vi "Module Loop.vi"(8 "error in (no error)":errorcluster, 11 "EStop Module in":refnum<class "EStop Module.lvclass">) -> (0 "error out":errorcluster, 3 "EStop Module out":refnum<class "EStop Module.lvclass">)   [LabVIEW 2020, in "VolatusControl.lvlib" / "EStop Module.lvclass"]
uses:
  EStop Module.lvclass
  C:/dev/lv20CE/relink/lv-volatus/Volatus/Module/Module.lvclass
  Volatus/Module/Module.lvclass
  Volatus/Module/Module.lvclass/Module.ctl
  <vilib>/Utility/error.llb/Error Cluster From Error Code.vi
  EStop Module.lvclass/EStop Module.ctl
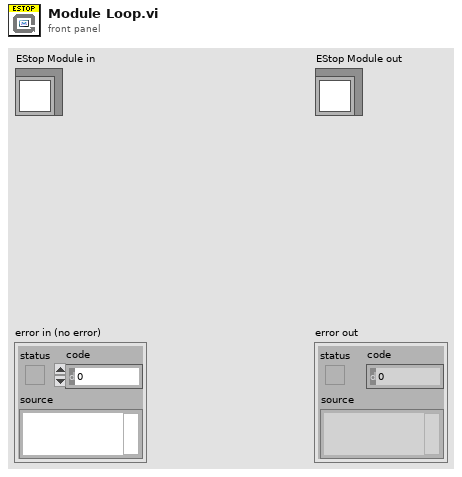
[diagram p1: front panel]
types:
  T1 = enum32{"Invalid", "Standard", "Closed", "Hidden", "Minimized", "Maximized"}
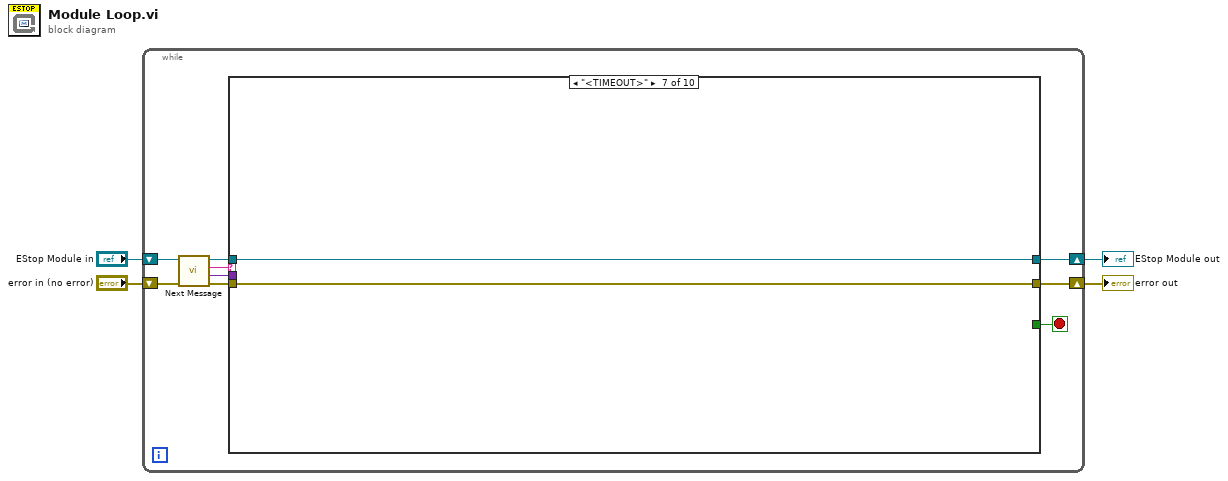
[diagram p0: block diagram]
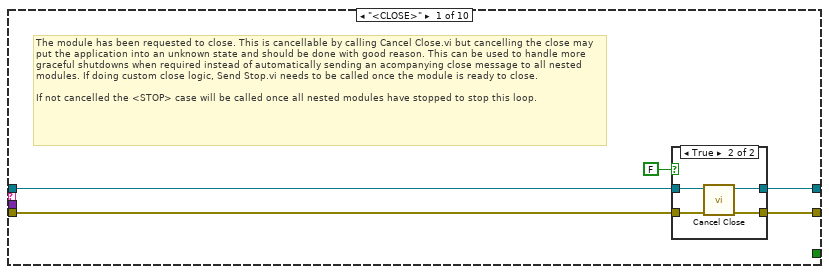
[diagram p2: hidden frame]
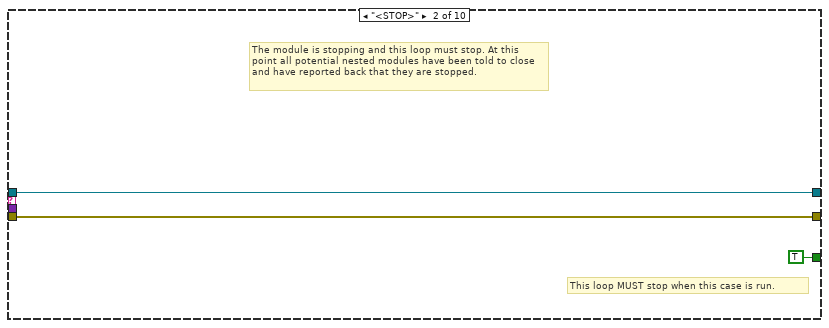
[diagram p4: hidden frame]
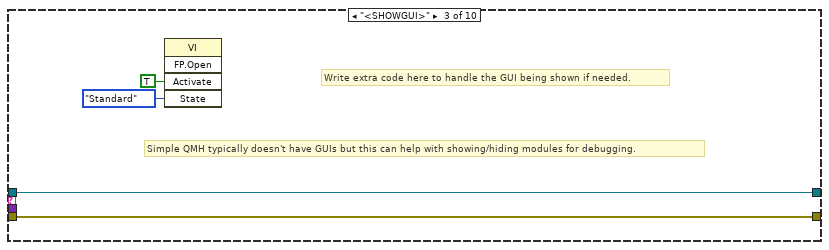
[diagram p5: hidden frame]
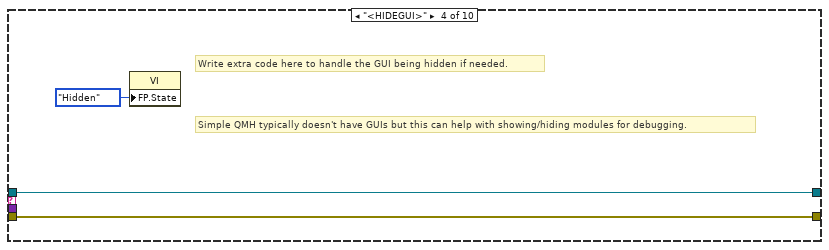
[diagram p6: hidden frame]
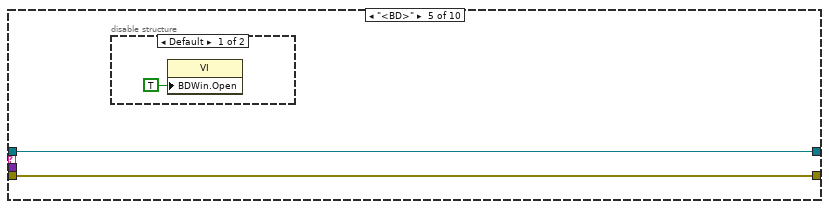
[diagram p7: hidden frame]
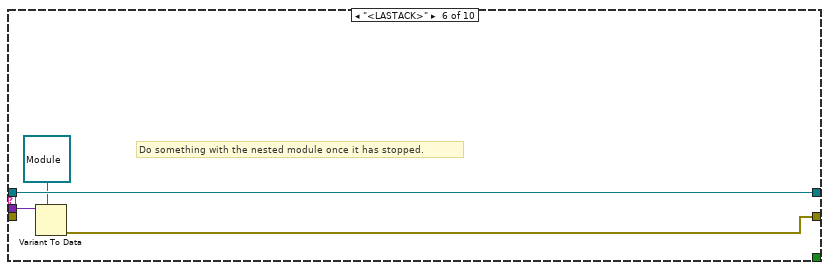
[diagram p9: hidden frame]
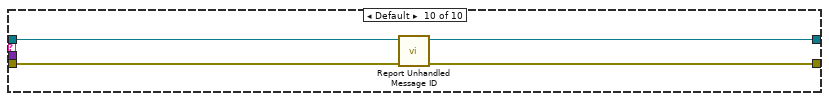
[diagram p12: hidden frame]
diagram:
  n1 = while {
    shift-right: [w8] -> w2
    shift-left: "EStop Module in" -> [w13]
    shift-right: [w7] -> w1
    shift-left: "error in (no error)" -> [w12]
    stop <- w6 stop-if-true
    n2 = call "Next Message.vi"("error in (no error)"=w12, "Module in"=w13) -> ("error out"=w11:errorcluster, "Data"=w5:variant, "ID"=w10:string, "Module out"=w9:refnum<class "EStop Module.lvclass">)  [unwired: 6 in]
    n3 = case shown="\"<TIMEOUT>\"" w10 {
      tunnel: w11 -> [w18 w26 w30 w33 w35 _ w42 w44 w46 w51]
      tunnel: w9 -> [w16 w27 w31 w34 w36 w41 w43 w45 w47 w49]
      tunnel: [w15 w27 w31 w34 w36 w41 w43 w45 w47 w48] -> w8
      tunnel: [w17 w26 w30 w33 w35 w38 w42 w44 w46 w50] -> w7
      tunnel: [_ TRUE _ _ _ _ _ _ _ _] -> w6
      tunnel: w5 -> [_ _ _ _ _ w40 _ _ _ _]
      frame "<CLOSE>" {
        # "The module has been requested to close. This is cancellable by calling Cancel Close.vi but cancelling the close may put the application into an unknown state and should be done with good reason. This can be used to handle more graceful shutdowns when required instead of automatically sending an acompanying close message to all nested modules. If doing custom close logic, Send Stop.vi needs to be called once the module is ready to close.\n\nIf not cancelled the <STOP> case will be called once all nested modules have stopped to stop this loop."
        n4 = case shown="True" FALSE {
          tunnel: w18 -> [w19 w24]
          tunnel: [w19 w23] -> w17
          tunnel: w16 -> [w20 w22]
          tunnel: [w20 w21] -> w15
          frame False {
          }
          frame True {
            n5 = call "Cancel Close.vi"("error in (no error)"=w24, "Module in"=w22) -> ("error out"=w23:errorcluster, "Module out"=w21:refnum<class "EStop Module.lvclass">)  [unwired: 8 in]
          }
        }
      }
      frame "<STOP>" {
        # "This loop MUST stop when this case is run."
        # "The module is stopping and this loop must stop. At this point all potential nested modules have been told to close and have reported back that they are stopped."
      }
      frame "<SHOWGUI>" {
        # "Simple QMH typically doesn't have GUIs but this can help with showing/hiding modules for debugging."
        # "Write extra code here to handle the GUI being shown if needed."
        n6 = invoke class="VI" method="FP.Open"("Activate"=TRUE ("Activate?"), "State"=T1."Standard") -> ()  [unwired: 3 in, 5 out]
      }
      frame "<HIDEGUI>" {
        # "Simple QMH typically doesn't have GUIs but this can help with showing/hiding modules for debugging."
        # "Write extra code here to handle the GUI being hidden if needed."
        n7 = property class="VI"("FP.State"=T1."Hidden" ("Front Panel Window:State")) -> ()  [unwired: 2 in, 2 out]
      }
      frame "<BD>" {
        n8 = disable-structure shown="Default" {
          frame condition #0 (active) {
            n9 = property class="VI"("BDWin.Open"=TRUE ("Block Diagram Window:Open")) -> ()  [unwired: 2 in, 2 out]
          }
          frame condition #1 {
          }
        }
      }
      frame "<LASTACK>" {
        # "Do something with the nested module once it has stopped."
        n10 = Variant To Data(type=refnum<class "Module.lvclass"> refnum ("Volatus:Module"), Variant=w40) -> (error out=w38:errorcluster)  [unwired: 1 in, 1 out]
      }
      frame "<TIMEOUT>" {
      }
      frame "Initialize" {
      }
      frame "EStop" {
      }
      frame Default {
        n11 = call "Report Unhandled Message ID.vi"("error in (no error)"=w51, "Module in"=w49) -> ("error out"=w50:errorcluster, "Module out"=w48:refnum<class "EStop Module.lvclass">)  [unwired: 8 in]
      }
    }
  }
  "error out" <- w1
  "EStop Module out" <- w2
